vi "Formula_Node_Ejercicio.vi"() -> ()   [LabVIEW 2020]
panel:
  out "XY Graph":cluster{"X":dbl, "Y":dbl}[](graph)
  out "Waveform Graph":dbl[](graph)
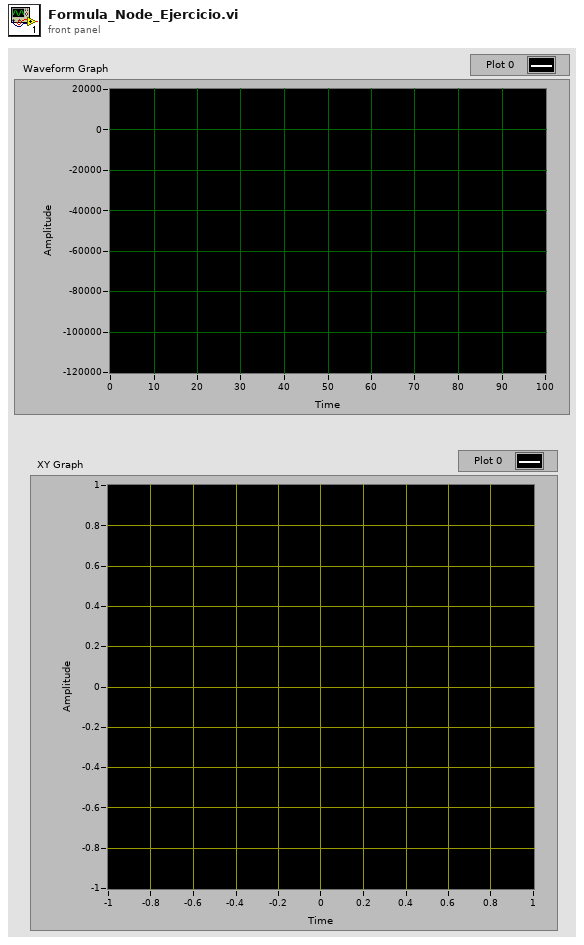
[diagram p1: front panel]
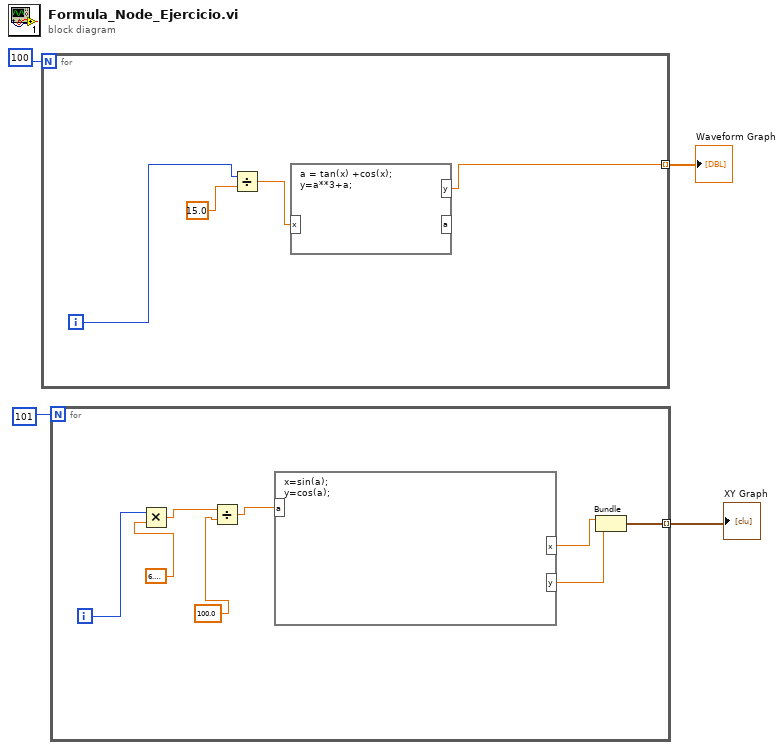
[diagram p0: block diagram]
diagram:
  n1 = for {
    N: 100 -> [_]
    tunnel: [w5] -> w4 mode=indexing
    i -> [w7]
    n2 = Divide(x=w7, y=15.0) -> (x/y=w6:dbl)
    n3 = formula code="a = tan(x) +cos(x);\ny=a**3+a;"("x"=w6) -> ("y"=w5:dbl)  [unwired: 1 out]
  }
  "Waveform Graph" <- w4
  n4 = for {
    N: 101 -> [_]
    tunnel: [w9] -> w1 mode=indexing
    i -> [w14]
    n5 = Multiply(x=w14, y=6.283185307179586) -> (x*y=w12:dbl)
    n6 = Divide(x=w12, y=100.0) -> (x/y=w10:dbl)
    n7 = formula code="x=sin(a);\ny=cos(a);"("a"=w10) -> ("x"=w16:dbl, "y"=w15:dbl)
    n8 = Bundle("x"=w16, "y"=w15) -> (w9:cluster{"x":dbl, "y":dbl})  [unwired: 1 in]
  }
  "XY Graph" <- w1
